vi "Split Commits.vi"(8 "error in":errorcluster, 10 "Commit String":string, 11 "Peer Review in":refnum<class "Peer Review.lvclass">) -> (0 "error out":errorcluster, 3 "Peer Review out":refnum<class "Peer Review.lvclass">)   [LabVIEW 2020, in "Peer Review.lvclass"]
uses:
  Peer Review.lvclass
  TypeDefs/Commit Info.ctl
  Peer Review.lvclass/Peer Review.ctl
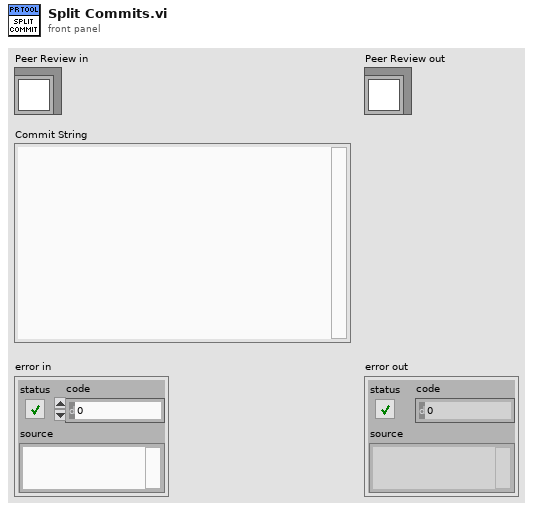
[diagram p1: front panel]
types:
  T1 = typedef "Peer Review.lvclass/Commit Info.ctl" = cluster{"Commit ID":i32, "Hash":string, "Merge Commit?":bool, "Merge Hash":string, "Author":string, "Time Stamp":timestamp, "Description":string, "File Count":i32, "File List":string[]}
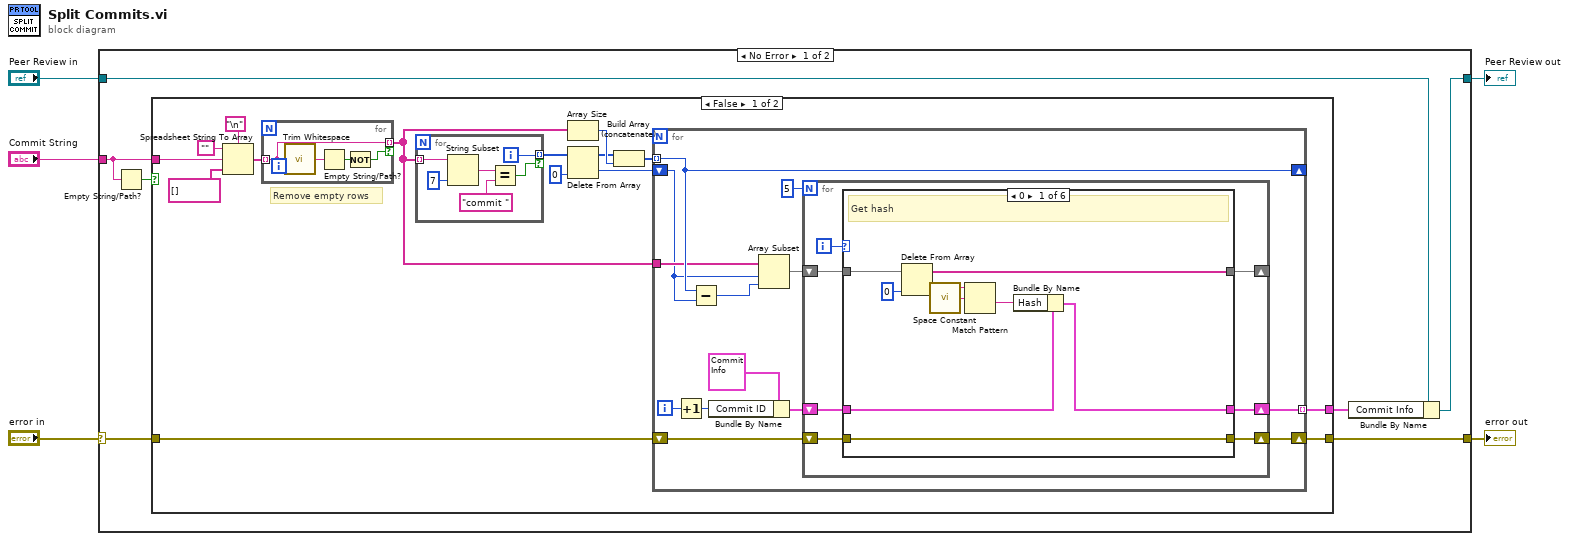
[diagram p0: block diagram]
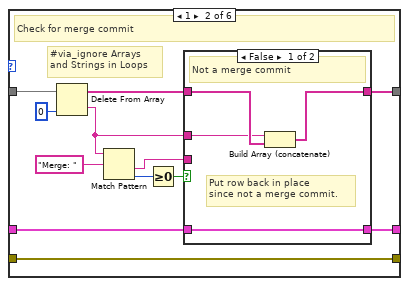
[diagram p2: hidden frame]
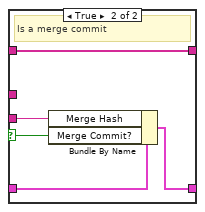
[diagram p3: hidden frame]
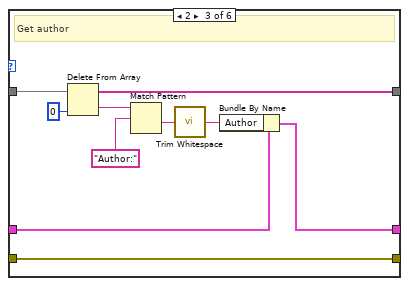
[diagram p4: hidden frame]
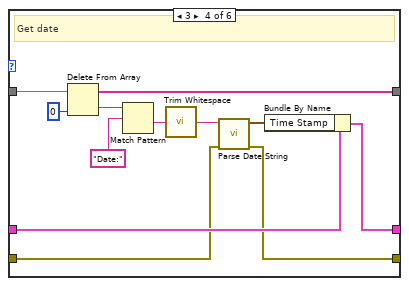
[diagram p5: hidden frame]
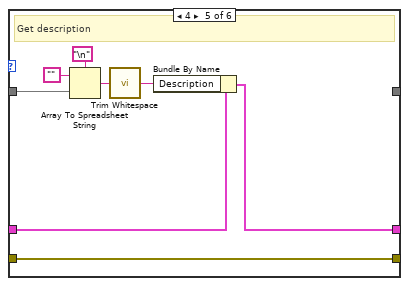
[diagram p6: hidden frame]
diagram:
  n1 = case shown="No Error" "error in" {
    selector: "error in" -> [w12 w122]
    tunnel: "Commit String" -> [w10 _]
    tunnel: [w11 w122] -> w3
    tunnel: "Peer Review in" -> [w7 w123]
    tunnel: [w6 w123] -> w1
    frame No Error {
      n2 = Empty String/Path?(string/path=w10) -> (empty?=w9:bool)
      n3 = case shown="False" w9 {
        tunnel: w12 -> [w16 w121]
        tunnel: [w15 w121] -> w11
        tunnel: w10 -> [w14 _]
        tunnel: [w13 _] -> w8
        frame False {
          # "Remove empty rows"
          n4 = Spreadsheet String To Array(delimiter (Tab)="\n" ("Line Feed Constant"), format string="", spreadsheet string=w14, array type (2D Dbl)=string[] []) -> (array=w18:string[])
          n5 = for {
            tunnel: w18 -> [w30] mode=indexing
            tunnel: [w30] -> w17 mode=indexing if=w28
            n6 = call <vilib>:"Trim Whitespace.vi"("string"=w30) -> ("trimmed string"=w31:string)  [unwired: 1 in]
            n7 = Empty String/Path?(string/path=w31) -> (empty?=w29:bool)
            n8 = Not(x=w29) -> (.not. x?=w28:bool)
          }
          n9 = for {
            tunnel: w17 -> [w120] mode=indexing
            tunnel: [w116] -> w19 mode=indexing if=w115
            i -> [w116]
            n10 = String Subset(string=w120, length (rest)=7 ("length (rest)")) -> (substring=w118:string)  [unwired: 1 in]
            n11 = Equal?(x=w118, y="commit " ("format string")) -> (x = y?=w115:bool)
          }
          n12 = Array Size(array=w17) -> (size(s)=w22:i32)
          n13 = Delete From Array(array=w19, index=0) -> (deleted portion=w23:i32, array with subset deleted=w21:i32[])  [unwired: 1 in]
          n14 = Build Array (concatenate)(w21, w22) -> (w20:i32[])
          n15 = for {
            shift-right: [w44] -> _
            shift-left: w23 -> [w42]
            tunnel: w20 -> [w44] mode=indexing
            tunnel: w17 -> [w43]
            tunnel: [w36] -> w13 mode=indexing
            shift-right: [w33] -> w15
            shift-left: w16 -> [w34]
            i -> [w35]
            n16 = Increment(x=w35) -> (x+1=w32:i32)
            n17 = Subtract(x=w44, y=w42) -> (x-y=w41:i32)
            n18 = Bundle By Name(cluster=T1 {"Commit ID"=0, "Hash"="", "Merge Commit?"=FALSE, "Merge Hash"="", "Author"="", "Time Stamp"=timestamp(0 s since 1904-01-01), "Description"="", "File Count"=0, "File List"=[]}, "Commit ID"=w32) -> (w39:T1)
            n19 = Array Subset(array=w43, index=w42, length=w41) -> (w38:string[])
            n20 = for {
              N: 5 -> [_]
              shift-right: [w49] -> _
              shift-left: w38 -> [w51]
              shift-right: [w47] -> w36
              shift-left: w39 -> [w48]
              shift-right: [w45] -> w33
              shift-left: w34 -> [w46]
              i -> [w50]
              n21 = case shown="0" w50 {
                tunnel: w51 -> [w59 w71 w90 w102 w106 w114]
                tunnel: [w58 w63 w89 w101 _ w114] -> w49
                tunnel: w48 -> [w57 w70 w88 w100 w111 w113]
                tunnel: [w56 w69 w87 w99 w110 w113] -> w47
                tunnel: w46 -> [w52 w61 w83 w94 w104 w112]
                tunnel: [w52 w61 w83 w93 w104 w112] -> w45
                frame 0 {
                  # "Get hash"
                  n22 = Delete From Array(array=w59, index=0) -> (deleted portion=w54:string, array with subset deleted=w58:string[])  [unwired: 1 in]
                  n23 = call <vilib>:"Space Constant.vi"() -> ("String"=w55:string)
                  n24 = Match Pattern(string=w54, regular expression=w55) -> (after substring=w53:string)  [unwired: 1 in, 3 out]
                  n25 = Bundle By Name(cluster=w57, "Hash"=w53) -> (w56:T1)
                }
                frame 1 {
                  # "#via_ignore Arrays and Strings in Loops"
                  # "Check for merge commit"
                  n26 = Delete From Array(array=w71, index=0) -> (deleted portion=w65:string, array with subset deleted=w64:string[])  [unwired: 1 in]
                  n27 = Match Pattern(string=w65, regular expression="Merge: ") -> (after substring=w62:string, offset past match=w67:i32)  [unwired: 1 in, 2 out]
                  n28 = Greater Or Equal To 0?(x=w67) -> (x >= 0?=w66:bool)
                  n29 = case shown="False" w66 {
                    selector: w66 -> [_ w79]
                    tunnel: w70 -> [w74 w81]
                    tunnel: [w74 w80] -> w69
                    tunnel: w65 -> [w73 _]
                    tunnel: w64 -> [w76 w77]
                    tunnel: [w75 w77] -> w63
                    tunnel: w62 -> [_ w78]
                    frame False {
                      # "Put row back in place\nsince not a merge commit."
                      # "Not a merge commit"
                      n30 = Build Array (concatenate)(w73, w76) -> (w75:string[])
                    }
                    frame True {
                      # "Is a merge commit"
                      n31 = Bundle By Name(cluster=w81, "Merge Hash"=w78, "Merge Commit?"=w79) -> (w80:T1)
                    }
                  }
                }
                frame 2 {
                  # "Get author"
                  n32 = Delete From Array(array=w90, index=0) -> (deleted portion=w86:string, array with subset deleted=w89:string[])  [unwired: 1 in]
                  n33 = Match Pattern(string=w86, regular expression="Author:") -> (after substring=w85:string)  [unwired: 1 in, 3 out]
                  n34 = call <vilib>:"Trim Whitespace.vi"("string"=w85) -> ("trimmed string"=w82:string)  [unwired: 1 in]
                  n35 = Bundle By Name(cluster=w88, "Author"=w82) -> (w87:T1)
                }
                frame 3 {
                  # "Get date"
                  n36 = Delete From Array(array=w102, index=0) -> (deleted portion=w98:string, array with subset deleted=w101:string[])  [unwired: 1 in]
                  n37 = Match Pattern(string=w98, regular expression="Date:") -> (after substring=w96:string)  [unwired: 1 in, 3 out]
                  n38 = call <vilib>:"Trim Whitespace.vi"("string"=w96) -> ("trimmed string"=w92:string)  [unwired: 1 in]
                  n39 = call "Parse Date String.vi"("error in"=w94, "Date String"=w92) -> ("error out"=w93:errorcluster, "Time Stamp"=w95:timestamp)  [unwired: 8 in]
                  n40 = Bundle By Name(cluster=w100, "Time Stamp"=w95) -> (w99:T1)
                }
                frame 4 {
                  # "Get description"
                  n41 = Array To Spreadsheet String(delimiter (Tab)="\n" ("Line Feed Constant"), array=w106, 3:"" ("format string")) -> (spreadsheet string=w109:string)
                  n42 = call <vilib>:"Trim Whitespace.vi"("string"=w109) -> ("trimmed string"=w105:string)  [unwired: 1 in]
                  n43 = Bundle By Name(cluster=w111, "Description"=w105) -> (w110:T1)
                }
                frame Default {
                  # "Invalid case"
                }
              }
            }
          }
        }
        frame True {
        }
      }
      n44 = Bundle By Name(cluster=w7, "Commit Info"=w8) -> (w6:refnum<class "Peer Review.lvclass">)
    }
    frame Error {
    }
  }
  "error out" <- w3
  "Peer Review out" <- w1
